vi "ShowCompiled.vi"(1 "States":string[](array[string]), 2 "Durations":dbl[](array[numeric])) -> (0 "Digital Waveform Graph":digitaldata(graph))   [LabVIEW 2014]
uses:
  <vilib>/Waveform/DTblOps.llb/DTbl Spreadsheet String to Digital.vi
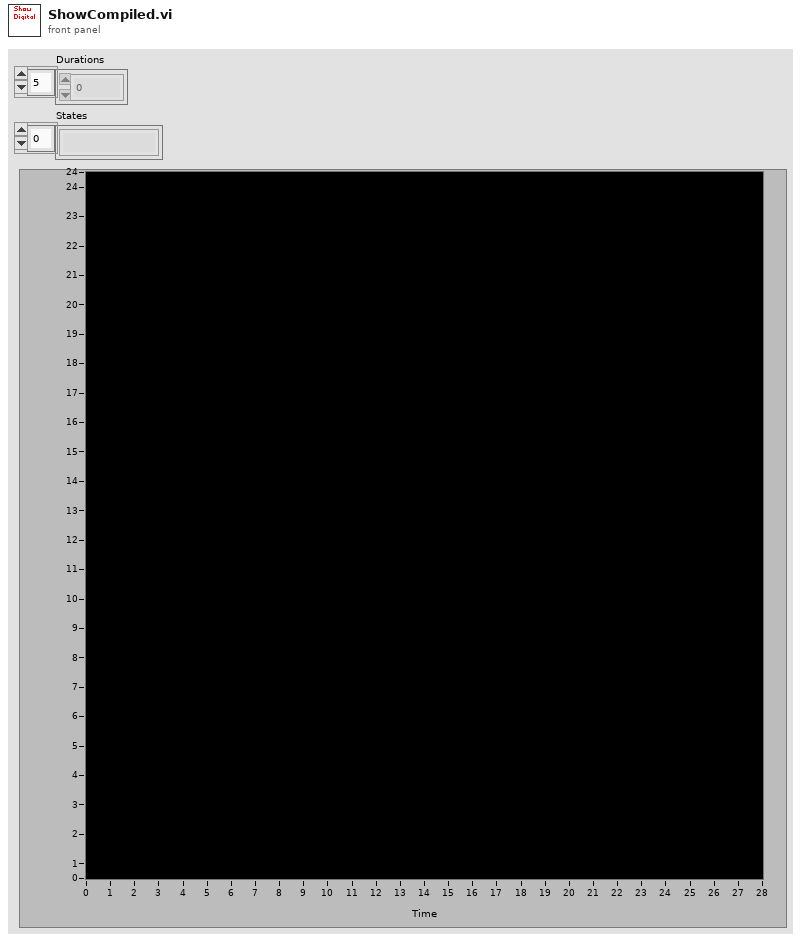
[diagram p1: front panel]
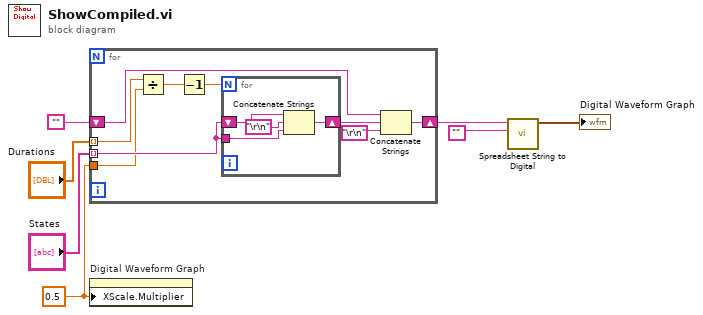
[diagram p0: block diagram]
diagram:
  w3 = 0.5 ("y")
  n1 = for {
    tunnel: "Durations" -> [w11] mode=indexing
    tunnel: "States" -> [w16] mode=indexing
    shift-right: [w13] -> w4
    shift-left: "" -> [w14]
    tunnel: w3 -> [w9]
    n2 = Divide(x=w11, y=w9) -> (x/y=w10:dbl)
    n3 = Decrement(x=w10) -> (x-1=w8:dbl)
    n4 = for {
      N: w8 -> [_]
      shift-right: [w19] -> w15
      shift-left: w16 -> [w18]
      tunnel: w16 -> [w20]
      n5 = Concatenate Strings(w18, "\r\n", w20) -> (w19:string)
    }
    n6 = Concatenate Strings(w14, w15, "\r\n") -> (w13:string)
  }
  n7 = property on="Digital Waveform Graph" class="DigitalGraph (strict)"("XScale.Multiplier"=w3) -> ()  [unwired: 2 in, 2 out]
  n8 = call-poly <vilib>:"Spreadsheet String to Digital.vi"("delimiter (tab)"="", "spreadsheet string"=w4) -> ("digital data"=→"Digital Waveform Graph":digitaldata)  [unwired: 8 in, 1 out]
